vi "751AngleToResistance.vi"(0 "180 deg resistance":dbl, 2 "0 deg resistance":dbl, 3 "Angle":dbl) -> (1 "Resistance":dbl)   [LabVIEW 2025]
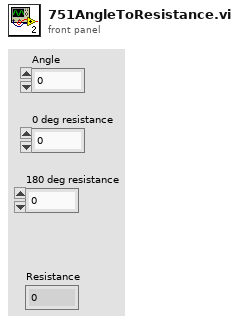
[diagram p1: front panel]
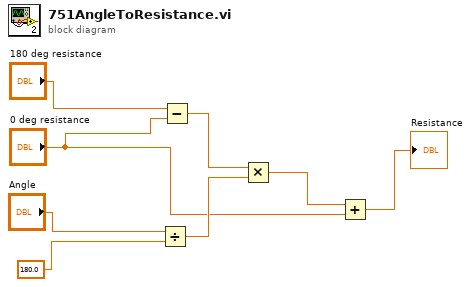
[diagram p0: block diagram]
diagram:
  n1 = Divide(x="Angle", y=180.0) -> (x/y=w5:dbl)
  n2 = Subtract(x="180 deg resistance", y="0 deg resistance") -> (x-y=w6:dbl)
  n3 = Multiply(x=w6, y=w5) -> (x*y=w3:dbl)
  n4 = Add(x=w3, y="0 deg resistance") -> (x+y=→"Resistance":dbl)
